vi "test.vi"() -> ()   [LabVIEW 2016]
panel:
  out "Console Out":string
  out "new picture":picture
  out "Version":string
  out "Tx Buffer":string
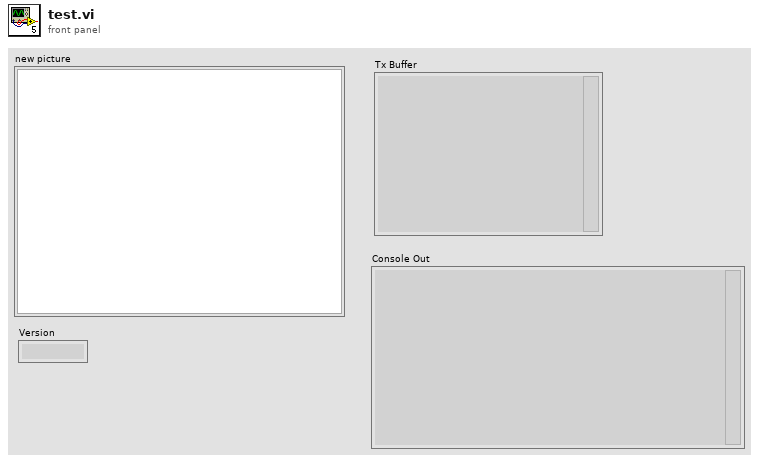
[diagram p1: front panel]
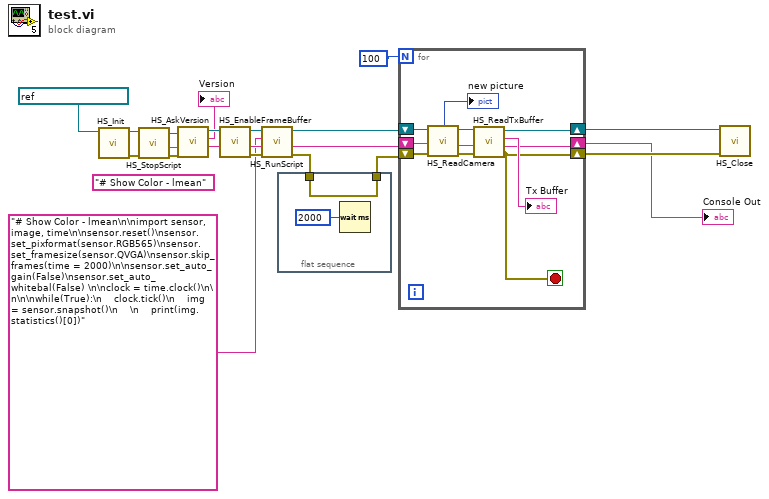
[diagram p0: block diagram]
diagram:
  (unwired) "# Show Color - lmean" ("script")
  n1 = call <userlib>:"HS_Init.vi"("VISA Refnum in"=refnum<visa-resource-name> "ASRL12::INSTR") -> ("error out"=w19:errorcluster, "VISA Refnum out"=w18:refnum<visa-resource-name>)  [unwired: 9 in]
  n2 = call <userlib>:"HS_StopScript.vi"("error in"=w19, "VISA Refnum in"=w18) -> ("error out"=w17:errorcluster, "Console Out"=w4:string, "VISA Refnum out"=w16:refnum<visa-resource-name>)  [unwired: 6 in, 1 out]
  n3 = call <userlib>:"HS_AskVersion.vi"("error in"=w17, "Console In"=w4, "VISA Refnum in"=w16) -> ("Console Out"=w14:string, "Version"=→"Version":string, "VISA Refnum out"=w15:refnum<visa-resource-name>)  [unwired: 5 in, 1 out]
  n4 = call <userlib>:"HS_EnableFrameBuffer.vi"("Console In"=w14, "VISA Refnum in"=w15) -> ("error out"=w12:errorcluster, "Console Out"=w11:string, "VISA Refnum out"=w10:refnum<visa-resource-name>)  [unwired: 6 in, 1 out]
  n5 = call <userlib>:"HS_RunScript.vi"("error in"=w12, "Console In"=w11, "script"="# Show Color - lmean\n\nimport sensor, image, time\n\nsensor.reset()\nsensor.set_pixformat(sensor.RGB565)\nsensor.set_framesize(sensor.QVGA)\nsensor.skip_frames(time = 2000)\n\nsensor.set_auto_gain(False)\nsensor.set_auto_whitebal(False) \n\nclock = time.clock()\n\n\n\nwhile(True):\n    clock.tick()\n    img = sensor.snapshot()\n    \n    print(img.statistics()[0])", "VISA Refnum in"=w10) -> ("error out"=w6:errorcluster, "Console Out"=w8:string, "VISA Refnum out"=w9:refnum<visa-resource-name>)  [unwired: 4 in, 1 out]
  n6 = flat-sequence {
    tunnel: [w22] -> w5
    tunnel: w6 -> [w22]
    frame #0 {
      n7 = Wait (ms)(milliseconds to wait=u32 2000) -> ()  [unwired: 1 out]
    }
  }
  n8 = for {
    N: 100 -> [_]
    shift-right: [w24] -> w2
    shift-left: w5 -> [w34]
    shift-right: [w30] -> w3
    shift-left: w9 -> [w33]
    shift-right: [w27] -> w1
    shift-left: w8 -> [w25]
    stop <- w24 stop-if-true
    n9 = call <userlib>:"HS_ReadCamera.vi"("error in"=w34, "Console In"=w25, "VISA Refnum in"=w33) -> ("error out"=w32:errorcluster, "Console Out"=w26:string, "VISA Refnum out"=w31:refnum<visa-resource-name>, "new picture"=→"new picture":picture)  [unwired: 1 in, 4 out]
    n10 = call <userlib>:"HS_ReadTxBuffer.vi"("error in"=w32, "Console In"=w26, "VISA Refnum in"=w31) -> ("error out"=w24:errorcluster, "Console Out"=w27:string, "Tx Buffer"=→"Tx Buffer":string, "VISA Refnum out"=w30:refnum<visa-resource-name>)  [unwired: 5 in]
  }
  "Console Out" <- w1
  n11 = call <userlib>:"HS_Close.vi"("error in (no error)"=w2, "VISA Refnum in"=w3) -> ()  [unwired: 10 in]
